vi "CallFetch.vi"(7 "Close?":bool, 8 "error in (no error)":errorcluster, 11 "reference":T1) -> (0 "error out":errorcluster, 1 "SRList":T2 {"SR#" format="%#_10g"}, 2 "DataValid?":bool)   [LabVIEW 2017, in "Server.lvlib" / "Oracle.lvlib"]
uses:
  Oracle.lvlib
  TypeDefs/SR List.ctl
  TypeDefs/SR Data.ctl
  <vilib>/addons/database/Connection.llb/Conn ObjectReference.ctl
  Server.lvlib
  <vilib>/addons/database/NI_Database_API.lvlib
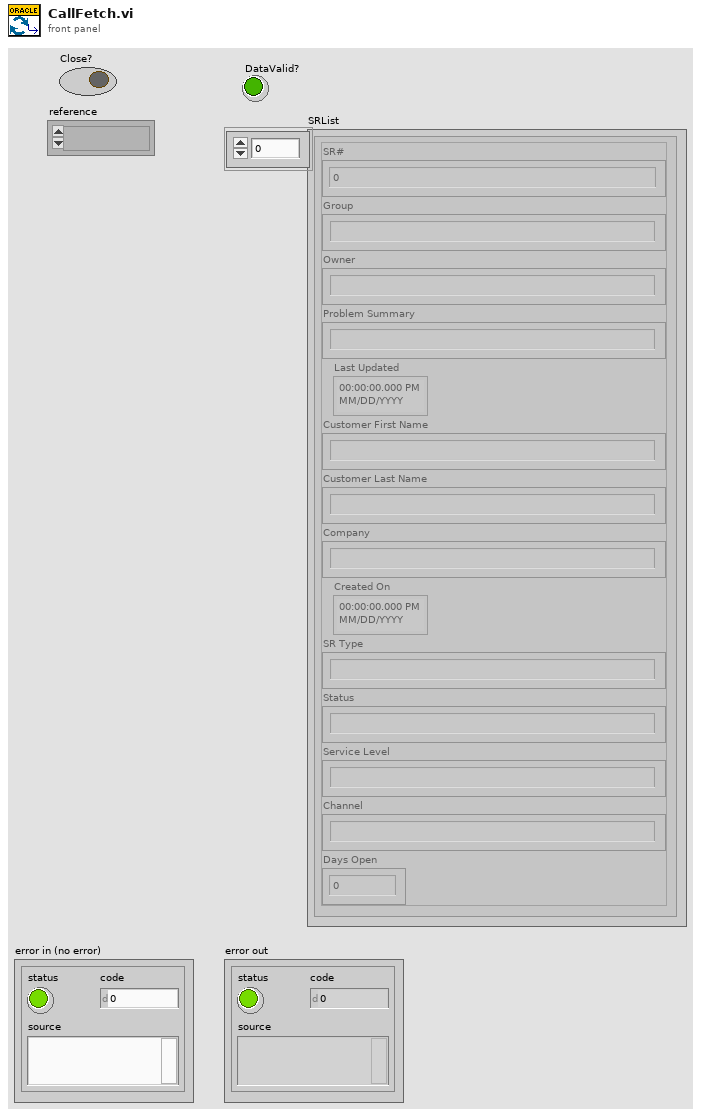
[diagram p1: front panel]
types:
  T1 = typedef "NI_Database_API.lvlib/Conn ObjectReference.ctl" = refnum<k1>
  T2 = typedef "Server.lvlib/SR List.ctl" = T3[]
  T3 = typedef "Server.lvlib/SR Data.ctl" = cluster{"SR#":dbl, "Group":string, "Owner":string, "Problem Summary":string, "Last Updated":timestamp, "Customer First Name":string, "Customer Last Name":string, "Company":string, "Created On":timestamp, "SR Type":string, "Status":string, "Service Level":string, "Channel":string, "Days Open":dbl}
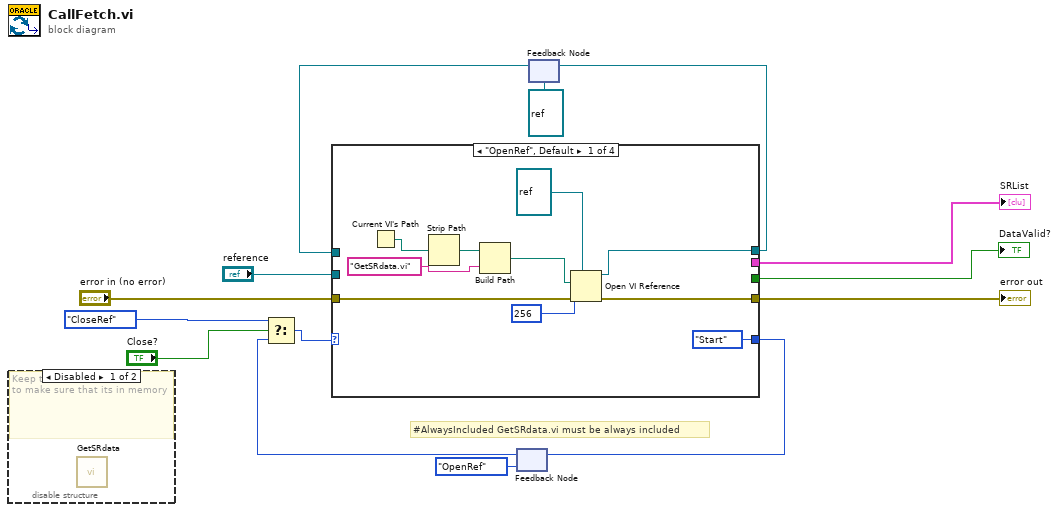
[diagram p0: block diagram]
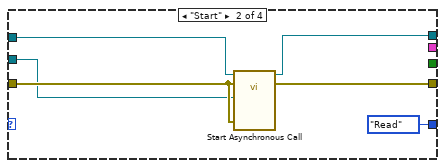
[diagram p2: hidden frame]
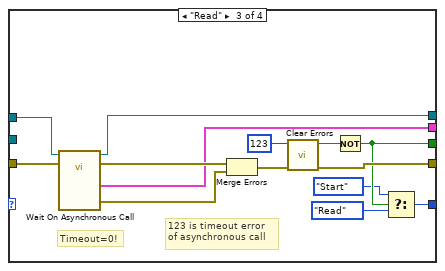
[diagram p3: hidden frame]
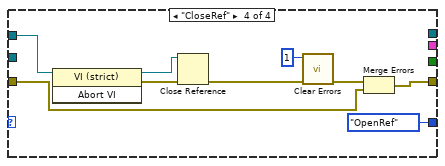
[diagram p4: hidden frame]
diagram:
  # "#AlwaysIncluded GetSRdata.vi must be always included"
  n1 = disable-structure shown="Disabled" {
    frame Disabled {
      # "Keep this VI here disabled \nto make sure that its in memory"
      n2 = call "GetSRdata.vi"() -> ()  [unwired: 10 in, 2 out]
    }
    frame Enabled {
    }
  }
  n3 = feedback #1(enum16{"OpenRef", "Start", "Read", "CloseRef"}."OpenRef") -> (w9:enum16{"OpenRef", "Start", "Read", "CloseRef"})
  n4 = Select(t=enum16{"OpenRef", "Start", "Read", "CloseRef"}."CloseRef", s="Close?", f=w9) -> (s? t:f=w7:enum16{"OpenRef", "Start", "Read", "CloseRef"})
  n5 = feedback #2(refnum<vi> refnum ("type specifier VI Refnum (for type only)")) -> (w4:refnum<vi>)
  n6 = case shown="\"OpenRef\", Default" w7 {
    tunnel: [w23 w30 w38 w46] -> w13
    tunnel: "error in (no error)" -> [w24 w29 w44 w45]
    tunnel: [_ _ w39 _] -> w12
    tunnel: [_ _ w35 _] -> w14
    tunnel: [enum16{"OpenRef", "Start", "Read", "CloseRef"}."Start" enum16{"OpenRef", "Start", "Read", "CloseRef"}."Read" w32 enum16{"OpenRef", "Start", "Read", "CloseRef"}."OpenRef" ("t")] -> w10
    tunnel: w4 -> [_ w28 w36 w51]
    tunnel: "reference" -> [_ w26 _ _]
    tunnel: [w19 w25 w31 _] -> w2
    frame "OpenRef", Default {
      n7 = Current VI's Path() -> (path=w18:path)
      n8 = Strip Path(path=w18) -> (stripped path=w16:path)  [unwired: 1 out]
      n9 = Build Path(base path=w16, name or relative path="GetSRdata.vi") -> (appended path=w17:path)
      n10 = Open VI Reference(type specifier VI Refnum (for type only)=refnum<vi> refnum, vi path=w17, options=256, error in (no error)=w24) -> (vi reference=w19:refnum<vi>, error out=w23:errorcluster)  [unwired: 2 in]
    }
    frame "Start" {
      n11 = call-by-ref "Start Asynchronous Call"(reference=w28, error in=w29, "Error In"=w29, "reference"=w26) -> (reference out=w25:refnum<vi>, error out=w30:errorcluster)  [unwired: 8 in, 2 out]
    }
    frame "Read" {
      # "123 is timeout error\nof asynchronous call"
      # "Timeout=0!"
      n12 = call-by-ref "Wait On Asynchronous Call"(reference=w36, error in=w44) -> (reference out=w31:refnum<vi>, error out=w43:errorcluster, "Error Out"=w40:errorcluster, "SRList"=w39:T2)  [unwired: 10 in]
      n13 = Merge Errors(w43, w40) -> (w41:errorcluster)
      n14 = call <vilib>:"Clear Errors.vi"("error in (no error)"=w41, "specific error code to clear (0: all)"=123) -> ("error out"=w38:errorcluster, "specific error cleared?"=w37:bool)  [unwired: 4 in]
      n15 = Not(x=w37) -> (.not. x?=w35:bool)
      n16 = Select(t=enum16{"OpenRef", "Start", "Read", "CloseRef"}."Start", s=w35, f=enum16{"OpenRef", "Start", "Read", "CloseRef"}."Read") -> (s? t:f=w32:enum16{"OpenRef", "Start", "Read", "CloseRef"})
    }
    frame "CloseRef" {
      n17 = invoke class="VI (strict)" method="Abort VI"(reference=w51) -> (reference out=w49:refnum<vi>, error out=w52:errorcluster)  [unwired: 2 in, 1 out]
      n18 = Close Reference(reference=w49, error in (no error)=w52) -> (error out=w50:errorcluster)
      n19 = call <vilib>:"Clear Errors.vi"("error in (no error)"=w50, "specific error code to clear (0: all)"=1) -> ("error out"=w48:errorcluster)  [unwired: 4 in, 1 out]
      n20 = Merge Errors(w48, w45) -> (w46:errorcluster)
    }
  }
  "DataValid?" <- w14
  "error out" <- w13
  "SRList" <- w12
  n21 = feedback-in #1(w10) -> ()
  n22 = feedback-in #2(w2) -> ()
